vi "Initialize.vi"(8 "error in (no error)":errorcluster, 9 "Port":u16=40000, 10 "Mock Replies":string[](array[string]), 11 "Mock Sift Proxy Server in":refnum<class "Mock Sift Proxy Server.lvclass">) -> (0 "error out":errorcluster, 3 "Mock Sift Proxy Server out":refnum<class "Mock Sift Proxy Server.lvclass">)   [LabVIEW 2024, in "Mock Sift Proxy Server.lvclass"]
uses:
  Mock Sift Proxy Server.lvclass
  Mock Sift Proxy Server.lvclass/Mock Sift Proxy Server.ctl
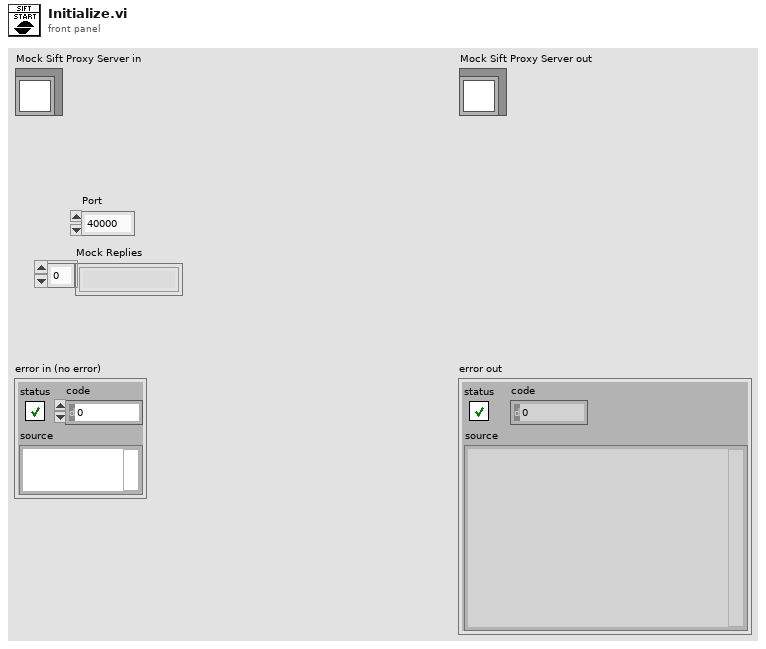
[diagram p1: front panel]
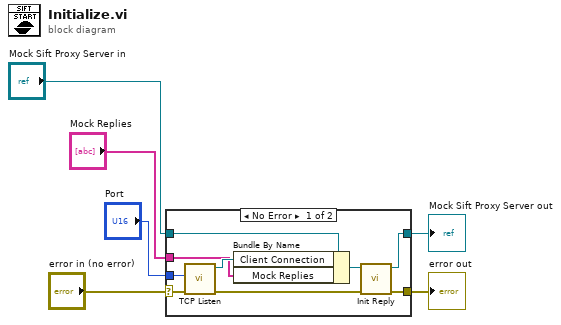
[diagram p0: block diagram]
diagram:
  n1 = case shown="No Error" "error in (no error)" {
    selector: "error in (no error)" -> [w13 w17]
    tunnel: [w10 w17] -> w5
    tunnel: [w7 w16] -> w3
    tunnel: "Mock Sift Proxy Server in" -> [w9 w16]
    tunnel: "Port" -> [w15 _]
    tunnel: "Mock Replies" -> [w12 _]
    frame No Error {
      n2 = call <vilib>:"TCP Listen.vi"("error in (no error)"=w13, "port"=w15) -> ("error out"=w11:errorcluster, "connection ID"=w14:refnum<k5>)  [unwired: 5 in, 3 out]
      n3 = Bundle By Name(cluster=w9, "Client Connection"=w14, "Mock Replies"=w12) -> (w8:refnum<class "Mock Sift Proxy Server.lvclass">)
      n4 = call-dynamic "Init Reply.vi"("error in (no error)"=w11, "Mock Sift Proxy Server in"=w8) -> ("error out"=w10:errorcluster, "Mock Sift Proxy Server out"=w7:refnum<class "Mock Sift Proxy Server.lvclass">)  [unwired: 8 in]
    }
    frame Error {
    }
  }
  "error out" <- w5
  "Mock Sift Proxy Server out" <- w3
